vi "UARTSendRec.vi"(0 "VISA resource name in":refnum<visa-resource-name>, 1 "Read Data Ref":refnum<vi>, 5 "H2F Frame Ref":refnum<vi>, 7 "Send LED Ref":refnum<vi>, 9 "Rec LED Ref":refnum<vi>, 11 "error in (no error)":errorcluster) -> (4 "VISA resource name out":refnum<visa-resource-name>, 8 "Recieved Data":T1, 10 "UART written count":u32, 15 "error out":errorcluster)   [LabVIEW 2018]
uses:
  TypeDefs/recDataClust.ctl
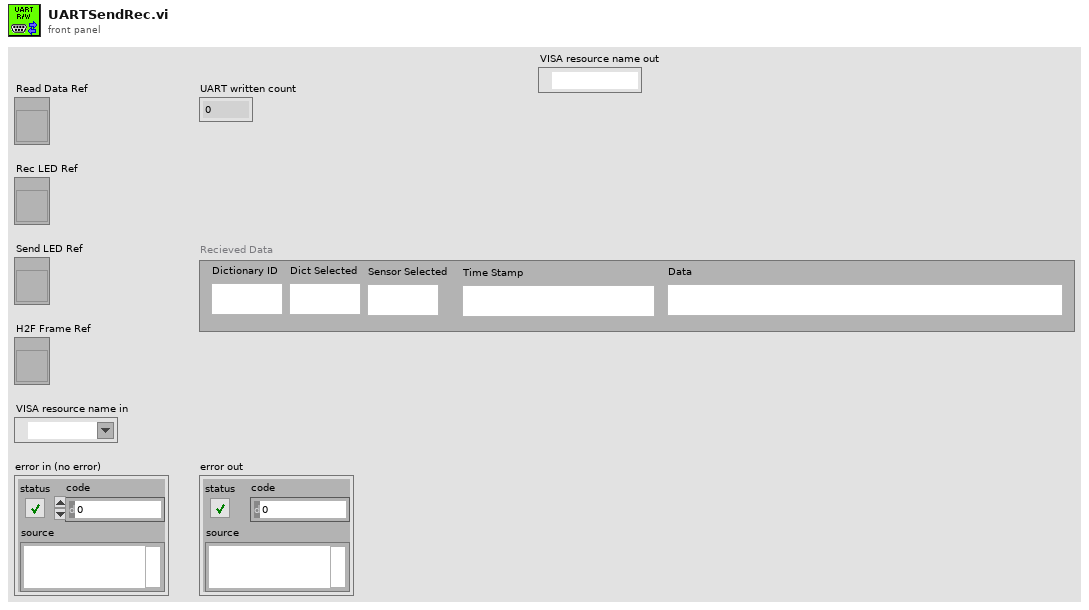
[diagram p1: front panel]
types:
  T1 = typedef "recDataClust.ctl" = cluster{"Dictionary ID":string, "Dict Selected":string, "Sensor Selected":string, "Time Stamp":string, "Data":string}
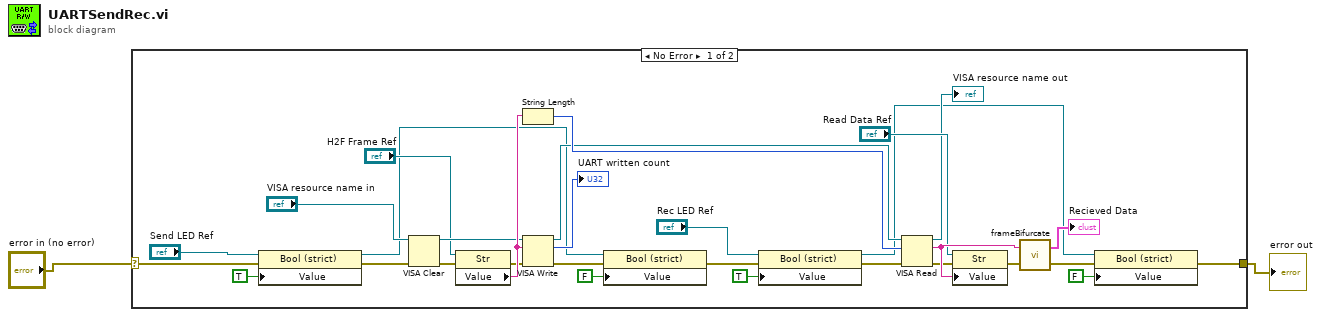
[diagram p0: block diagram]
diagram:
  n1 = case shown="No Error" "error in (no error)" {
    selector: "error in (no error)" -> [w3 w33]
    tunnel: [w9 w33] -> w2
    frame No Error {
      n2 = property on="Property Node" class="Bool (strict)"(reference="Send LED Ref", error in=w3, "Value"=TRUE ("Sending Command")) -> (reference out=w6:refnum<vi>, error out=w18:errorcluster)
      n3 = VISA Clear(VISA resource name="VISA resource name in", error in (no error)=w18) -> (VISA resource name out=w17:refnum<visa-resource-name>, error out=w16:errorcluster)
      n4 = property on="Property Node" class="Str"(reference="H2F Frame Ref", error in=w16) -> (error out=w14:errorcluster, "Value"=w24:string)  [unwired: 1 out]
      n5 = String Length(string=w24) -> (length=w25:i32)
      n6 = VISA Write(VISA resource name=w17, write buffer=w24, error in (no error)=w14) -> (VISA resource name out=w19:refnum<visa-resource-name>, return count=→"UART written count":u32, error out=w20:errorcluster)
      n7 = property on="Property Node" class="Bool (strict)"(reference=w6, error in=w20, "Value"=FALSE ("Sending Command")) -> (error out=w21:errorcluster)  [unwired: 1 out]
      n8 = property on="Property Node" class="Bool (strict)"(reference="Rec LED Ref", error in=w21, "Value"=TRUE ("Sending Command")) -> (reference out=w4:refnum<vi>, error out=w23:errorcluster)
      n9 = VISA Read(VISA resource name=w19, byte count=w25, error in (no error)=w23) -> (VISA resource name out=→"VISA resource name out":refnum<visa-resource-name>, read buffer=w30:string, error out=w28:errorcluster)  [unwired: 1 out]
      n10 = property on="Property Node" class="Str"(reference="Read Data Ref", error in=w28, "Value"=w30) -> (error out=w29:errorcluster)  [unwired: 1 out]
      n11 = call "frameBifurcate.vi"("error in (no error)"=w29, "H2F Frame"=w30) -> ("error out"=w10:errorcluster, "Bifurcated Recieved Data"=→"Recieved Data":T1)
      n12 = property on="Property Node" class="Bool (strict)"(reference=w4, error in=w10, "Value"=FALSE ("Sending Command")) -> (error out=w9:errorcluster)  [unwired: 1 out]
    }
    frame Error {
    }
  }
  "error out" <- w2
